vi "closeDevice.vi"(8 "error in (no error)":errorcluster, 10 "deviceName":string, 11 "AtomChipHWC in":refnum<class "AtomChipHWC.lvclass">) -> (0 "error out":errorcluster, 3 "AtomChipHWC out":refnum<class "AtomChipHWC.lvclass">)   [LabVIEW 2009, in "Hardware.lvlib" / "HWControllers.lvlib" / "AtomChipHWC.lvclass"]
doc: "Shut down a device, so it is no longer in use by labview."
uses:
  AtomChipHWC.lvclass
  AtomChipHWC.lvclass/AtomChipHWC.ctl
  Channels/Digital/DigitalOutput.lvclass
  Channels/VoltOutput/AnalogOutput.lvclass
  IntegrationManagement/CameraManager.lvclass
  Channels/DDSOutput/Generic/DDSOutput.lvclass
  Network Controllers/NetworkCamera/NetworkCamera.lvclass
  Network Controllers/CameraNetworkController/CameraNetworkController.lvclass
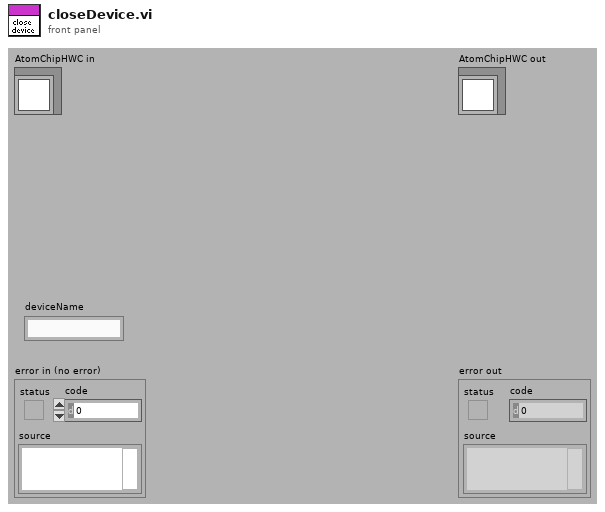
[diagram p1: front panel]
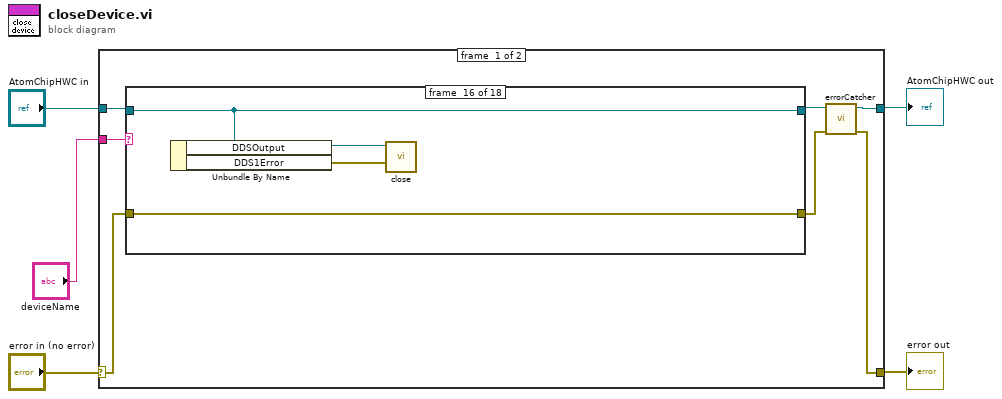
[diagram p0: block diagram]
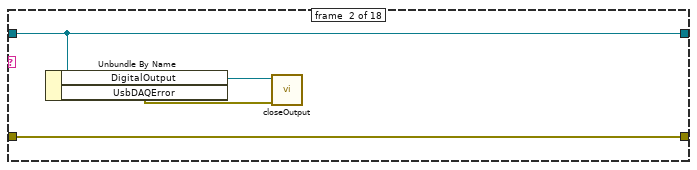
[diagram p3: hidden frame]
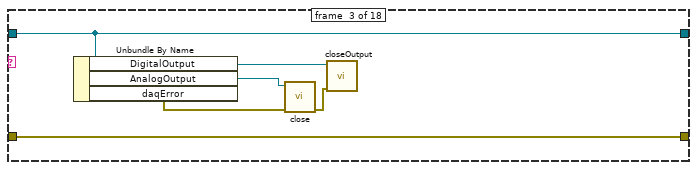
[diagram p4: hidden frame]
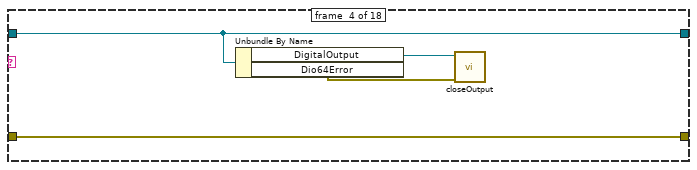
[diagram p5: hidden frame]
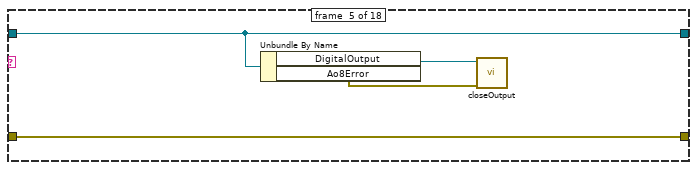
[diagram p6: hidden frame]
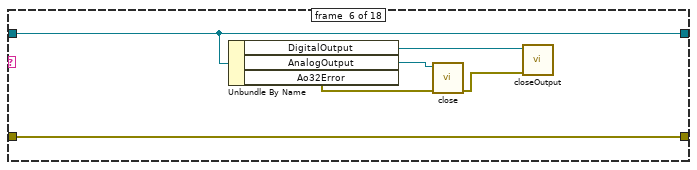
[diagram p7: hidden frame]
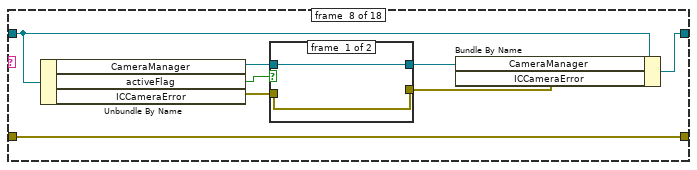
[diagram p9: hidden frame]
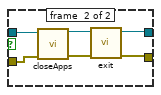
[diagram p10: hidden frame]
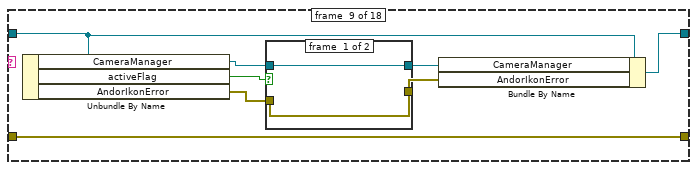
[diagram p11: hidden frame]
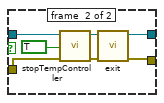
[diagram p12: hidden frame]
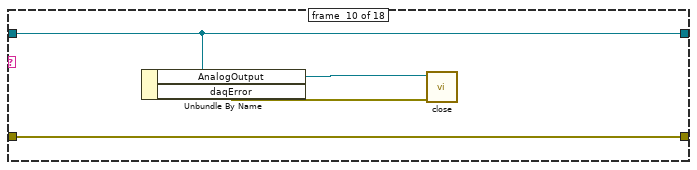
[diagram p13: hidden frame]
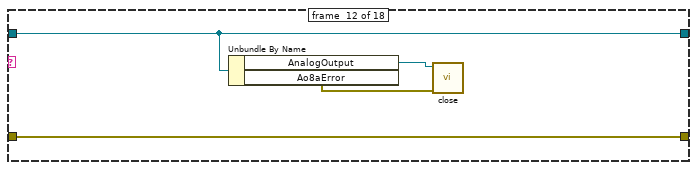
[diagram p15: hidden frame]
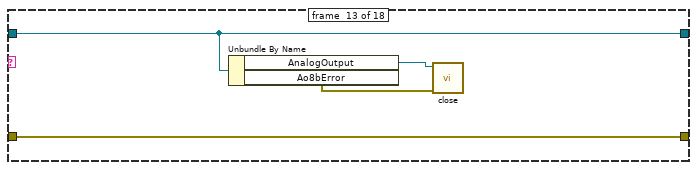
[diagram p16: hidden frame]
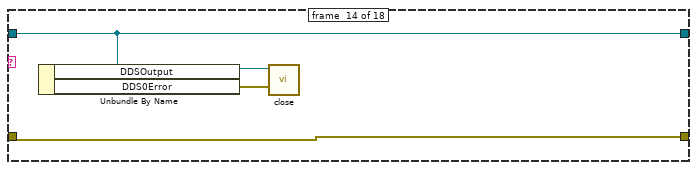
[diagram p17: hidden frame]
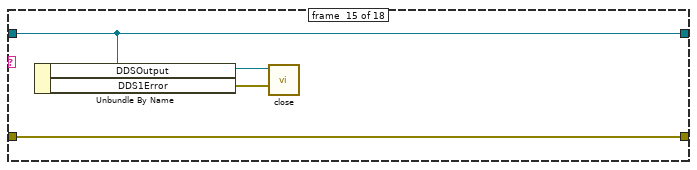
[diagram p18: hidden frame]
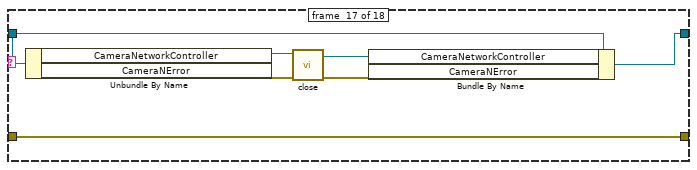
[diagram p19: hidden frame]
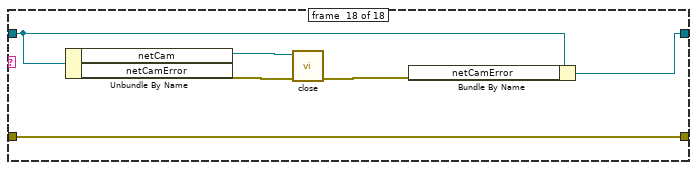
[diagram p20: hidden frame]
diagram:
  n1 = case shown="No Error" "error in (no error)" {
    selector: "error in (no error)" -> [w11 w114]
    tunnel: [w8 w114] -> w4
    tunnel: [w6 w113] -> w2
    tunnel: "AtomChipHWC in" -> [w12 w113]
    tunnel: "deviceName" -> [w10 _]
    frame #0 {
      n2 = case shown="\"Pixelfly\", \"ProEM_WinX32\"" w10 {
        tunnel: w12 -> [w14 w18 w23 w27 w31 w37 w40 w46 w62 w77 w79 w83 w87 w90 w94 w98 w105 w112]
        tunnel: [w14 w18 w23 w27 w31 w37 w40 w48 w64 w77 w79 w83 w87 w90 w94 w98 w103 w111] -> w7
        tunnel: w11 -> [w13 w15 w19 w25 w29 w33 w39 w42 w57 w74 w78 w80 w84 w88 w92 w96 w100 w110]
        tunnel: [w13 w15 w19 w25 w29 w33 w39 w42 w57 w74 w78 w80 w84 w88 w92 w96 w100 w110] -> w9
        frame #0 {
        }
        frame #1 {
          n3 = Unbundle By Name(w18) -> ("DigitalOutput"=w17:refnum<class "DigitalOutput.lvclass">, "UsbDAQError"=w16:errorcluster)
          n4 = call-dynamic "closeOutput.vi"("error in (no error)"=w16, "DigitalOutput in"=w17) -> ()  [unwired: 9 in, 1 out]
        }
        frame #2 {
          n5 = Unbundle By Name(w23) -> ("DigitalOutput"=w24:refnum<class "DigitalOutput.lvclass">, "AnalogOutput"=w22:refnum<class "AnalogOutput.lvclass">, "daqError"=w20:errorcluster)
          n6 = call-dynamic "close.vi"("error in (no error)"=w20, "AnalogOutput in"=w22) -> ("error out"=w21:errorcluster)  [unwired: 9 in]
          n7 = call-dynamic "closeOutput.vi"("error in (no error)"=w21, "DigitalOutput in"=w24) -> ()  [unwired: 9 in, 1 out]
        }
        frame #3 {
          n8 = Unbundle By Name(w27) -> ("DigitalOutput"=w28:refnum<class "DigitalOutput.lvclass">, "Dio64Error"=w26:errorcluster)
          n9 = call-dynamic "closeOutput.vi"("error in (no error)"=w26, "DigitalOutput in"=w28) -> ()  [unwired: 9 in, 1 out]
        }
        frame #4 {
          n10 = Unbundle By Name(w31) -> ("DigitalOutput"=w32:refnum<class "DigitalOutput.lvclass">, "Ao8Error"=w30:errorcluster)
          n11 = call-dynamic "closeOutput.vi"("error in (no error)"=w30, "DigitalOutput in"=w32) -> ()  [unwired: 9 in, 1 out]
        }
        frame #5 {
          n12 = Unbundle By Name(w37) -> ("DigitalOutput"=w38:refnum<class "DigitalOutput.lvclass">, "AnalogOutput"=w36:refnum<class "AnalogOutput.lvclass">, "Ao32Error"=w34:errorcluster)
          n13 = call-dynamic "close.vi"("error in (no error)"=w34, "AnalogOutput in"=w36) -> ("error out"=w35:errorcluster)  [unwired: 9 in]
          n14 = call-dynamic "closeOutput.vi"("error in (no error)"=w35, "DigitalOutput in"=w38) -> ()  [unwired: 9 in, 1 out]
        }
        frame #6 {
        }
        frame #7 {
          n15 = Unbundle By Name(w46) -> ("CameraManager"=w45:refnum<class "CameraManager.lvclass">, "activeFlag"=w44:bool, "ICCameraError"=w43:errorcluster)
          n16 = case shown="True" w44 {
            tunnel: [w50 w56] -> w47
            tunnel: [w49 w55] -> w41
            tunnel: w45 -> [w50 w52]
            tunnel: w43 -> [w49 w51]
            frame #0 {
            }
            frame #1 {
              n17 = call "closeApps.vi"("error in (no error)"=w51, "CameraManager in"=w52) -> ("error out"=w54:errorcluster, "CameraManager out"=w53:refnum<class "CameraManager.lvclass">)  [unwired: 8 in]
              n18 = call-dynamic "exit.vi"("error in (no error)"=w54, "CameraManager in"=w53) -> ("error out"=w55:errorcluster, "CameraManager out"=w56:refnum<class "CameraManager.lvclass">)  [unwired: 8 in]
            }
          }
          n19 = Bundle By Name(cluster=w46, "CameraManager"=w47, "ICCameraError"=w41) -> (w48:refnum<class "AtomChipHWC.lvclass">)
        }
        frame #8 {
          n20 = Unbundle By Name(w62) -> ("CameraManager"=w61:refnum<class "CameraManager.lvclass">, "activeFlag"=w60:bool, "AndorIkonError"=w59:errorcluster)
          n21 = case shown="True" w60 {
            tunnel: [w66 w72] -> w63
            tunnel: [w65 w67] -> w58
            tunnel: w59 -> [w65 w68]
            tunnel: w61 -> [w66 w69]
            frame #0 {
            }
            frame #1 {
              n22 = call "stopTempController.vi"("error in (no error)"=w68, "releaseWhenReady"=TRUE, "CameraManager in"=w69) -> ("error out"=w71:errorcluster, "CameraManager out"=w70:refnum<class "CameraManager.lvclass">)  [unwired: 7 in]
              n23 = call-dynamic "exit.vi"("error in (no error)"=w71, "CameraManager in"=w70) -> ("error out"=w67:errorcluster, "CameraManager out"=w72:refnum<class "CameraManager.lvclass">)  [unwired: 8 in]
            }
          }
          n24 = Bundle By Name(cluster=w62, "CameraManager"=w63, "AndorIkonError"=w58) -> (w64:refnum<class "AtomChipHWC.lvclass">)
        }
        frame #9 {
          n25 = Unbundle By Name(w77) -> ("AnalogOutput"=w76:refnum<class "AnalogOutput.lvclass">, "daqError"=w75:errorcluster)
          n26 = call-dynamic "close.vi"("error in (no error)"=w75, "AnalogOutput in"=w76) -> ()  [unwired: 9 in, 1 out]
        }
        frame #10 {
        }
        frame #11 {
          n27 = Unbundle By Name(w83) -> ("AnalogOutput"=w82:refnum<class "AnalogOutput.lvclass">, "Ao8aError"=w81:errorcluster)
          n28 = call-dynamic "close.vi"("error in (no error)"=w81, "AnalogOutput in"=w82) -> ()  [unwired: 9 in, 1 out]
        }
        frame #12 {
          n29 = Unbundle By Name(w87) -> ("AnalogOutput"=w86:refnum<class "AnalogOutput.lvclass">, "Ao8bError"=w85:errorcluster)
          n30 = call-dynamic "close.vi"("error in (no error)"=w85, "AnalogOutput in"=w86) -> ()  [unwired: 9 in, 1 out]
        }
        frame #13 {
          n31 = Unbundle By Name(w90) -> ("DDSOutput"=w91:refnum<class "DDSOutput.lvclass">, "DDS0Error"=w89:errorcluster)
          n32 = call-dynamic "close.vi"("error in (no error)"=w89, "DDSOutput in"=w91) -> ()  [unwired: 9 in, 1 out]
        }
        frame #14 {
          n33 = Unbundle By Name(w94) -> ("DDSOutput"=w95:refnum<class "DDSOutput.lvclass">, "DDS1Error"=w93:errorcluster)
          n34 = call-dynamic "close.vi"("error in (no error)"=w93, "DDSOutput in"=w95) -> ()  [unwired: 9 in, 1 out]
        }
        frame #15 {
          n35 = Unbundle By Name(w98) -> ("DDSOutput"=w99:refnum<class "DDSOutput.lvclass">, "DDS1Error"=w97:errorcluster)
          n36 = call-dynamic "close.vi"("error in (no error)"=w97, "DDSOutput in"=w99) -> ()  [unwired: 9 in, 1 out]
        }
        frame #16 {
          n37 = Unbundle By Name(w105) -> ("CameraNetworkController"=w106:refnum<class "CameraNetworkController.lvclass">, "CameraNError"=w101:errorcluster)
          n38 = call "close.vi"("error in (no error)"=w101, "CameraNetworkController in"=w106) -> ("error out"=w102:errorcluster, "CameraNetworkController out"=w104:refnum<class "CameraNetworkController.lvclass">)  [unwired: 8 in]
          n39 = Bundle By Name(cluster=w105, "CameraNetworkController"=w104, "CameraNError"=w102) -> (w103:refnum<class "AtomChipHWC.lvclass">)
        }
        frame #17 {
          n40 = Unbundle By Name(w112) -> ("netCam"=w109:refnum<class "NetworkCamera.lvclass">, "netCamError"=w108:errorcluster)
          n41 = call-dynamic "close.vi"("error in (no error)"=w108, "NetworkCamera in"=w109) -> ("error out"=w107:errorcluster)  [unwired: 9 in]
          n42 = Bundle By Name(cluster=w112, "netCamError"=w107) -> (w111:refnum<class "AtomChipHWC.lvclass">)
        }
      }
      n43 = call-dynamic "errorCatcher.vi"("error in (no error)"=w9, "HWController in"=w7) -> ("error out"=w8:errorcluster, "HWController out"=w6:refnum<class "AtomChipHWC.lvclass">)  [unwired: 8 in]
    }
    frame #1 {
    }
  }
  "error out" <- w4
  "AtomChipHWC out" <- w2
